vi "ENPH 354 Assignment 3 - Q1.vi"() -> ()   [LabVIEW 2021]
panel:
  out "?":dbl
  out "?":string
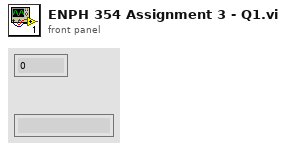
[diagram p1: front panel]
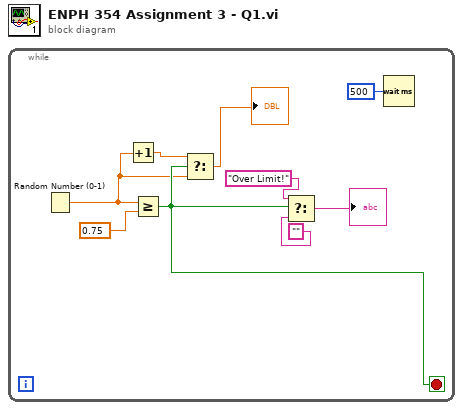
[diagram p0: block diagram]
diagram:
  n1 = while {
    stop <- w5 stop-if-true
    n2 = Random Number (0-1)() -> (number: 0 to 1=w2:dbl)
    n3 = Increment(x=w2) -> (x+1=w4:dbl)
    n4 = Greater Or Equal?(x=w2, y=0.75) -> (x >= y?=w5:bool)
    n5 = Select(t=w4, s=w5, f=w2) -> (s? t:f=→"?":dbl)
    n6 = Select(t="Over Limit!", s=w5, f="") -> (s? t:f=→"?":string)
    n7 = Wait (ms)(milliseconds to wait=u32 500) -> ()  [unwired: 1 out]
  }
